vi "bufferFileManager.vi"(0 "Base Path (C:\\)":path=path "C:/", 1 "Write Limit (6000 writes)":i32=6000, 2 "Number of Files (7)":i32=7, 3 "Mode (Use)":enum16{"Init", "Use"}(ring)=enum."Use", 5 "Data Byte String (empty string)":string, 9 "Header Byte String (empty string)":string, 11 "Error In (no error)":errorcluster caption="Error In (No Error)", 12 "File Name Template (BUFFER_)":string="BUFFER_", 13 "File Extension (none)":string) -> (4 "refnums":refnum<file>[](array[refnum]), 6 "File Index":i32, 10 "Write Index":i32, 15 "Error Out":errorcluster)   [LabVIEW 2020]
doc: "This function manages a disk buffer located at the \"Base Path\". The number of buffer files is set by the \"Number of Files\" input, and they are labeled BUFFER_X by default where X is the zero-based buffer file number. BUFFER_ can be replaced in the file name by the user-specified \"File Name Template\". For each call to this function the \"Byte String\" data is written to the buffer files in turn. Files are created, cleared, and switched to as needed when the buffer \"Write Limit\" is met. If \"Byte String\" is empty nothing is written and the write counter is not incremented. To ignore the write limit or number of file limit, set these values to equal -1."
panel:
  # "NOTE: Mode is not necessary for use so it is disabled."
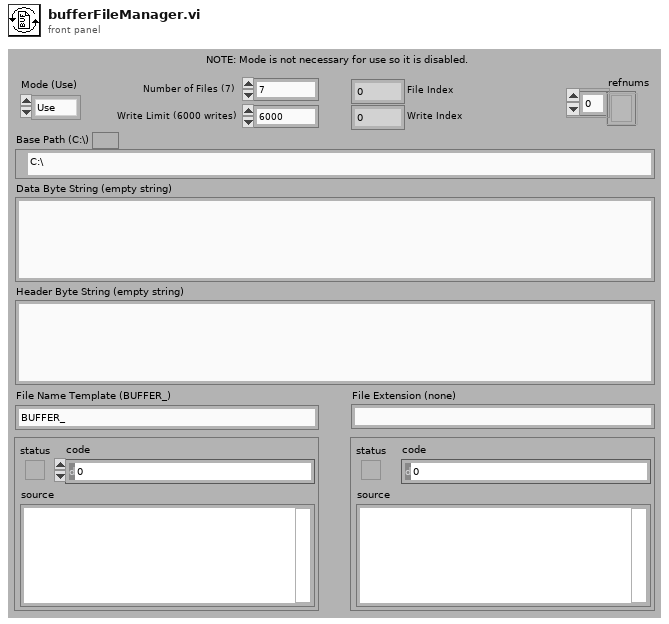
[diagram p1: front panel]
types:
  T1 = enum16{"open", "replace", "create", "open or create", "replace or create", "replace or create with confirmation"}
  T2 = cluster{"refnums":refnum<file>[], "File Index":i32, "Write Index":i32}
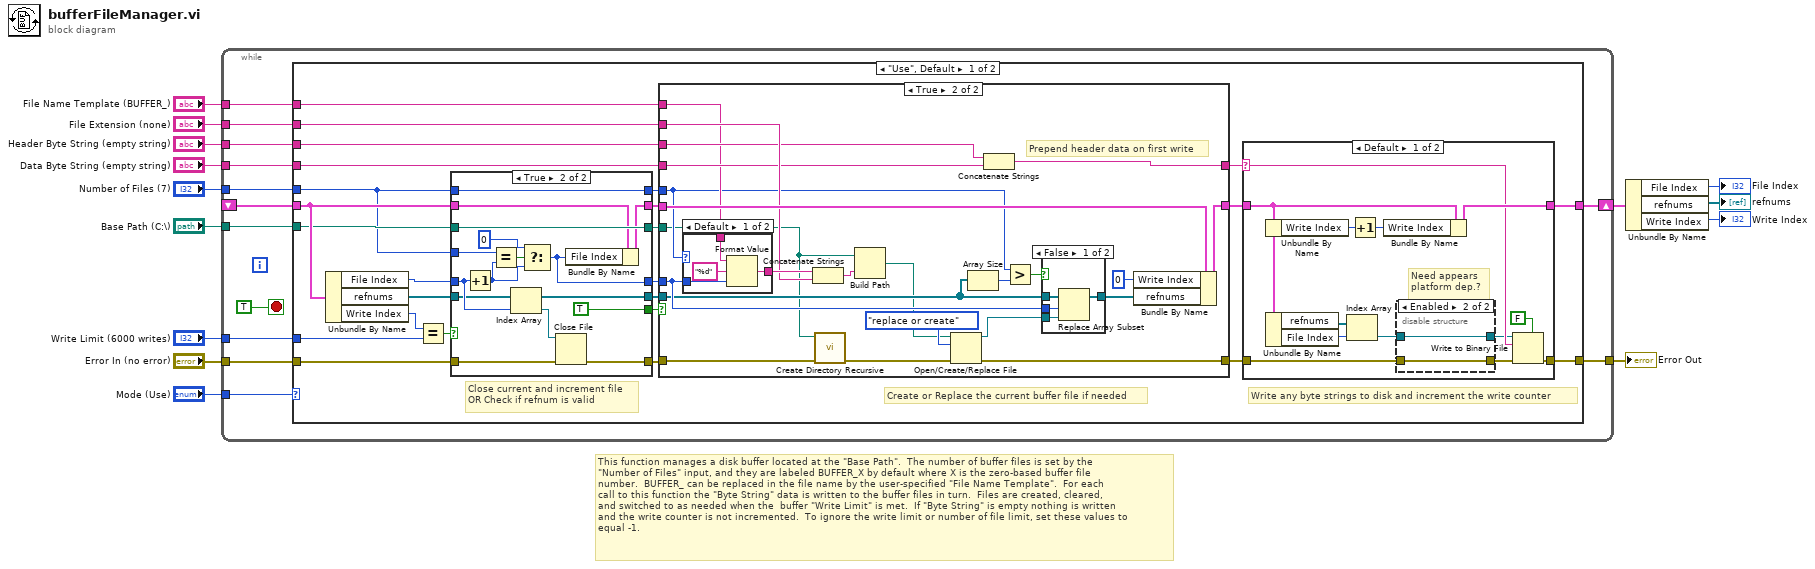
[diagram p0: block diagram]
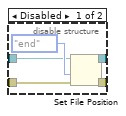
[diagram p2: hidden frame]
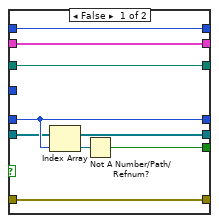
[diagram p4: hidden frame]
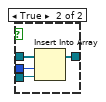
[diagram p7: hidden frame]
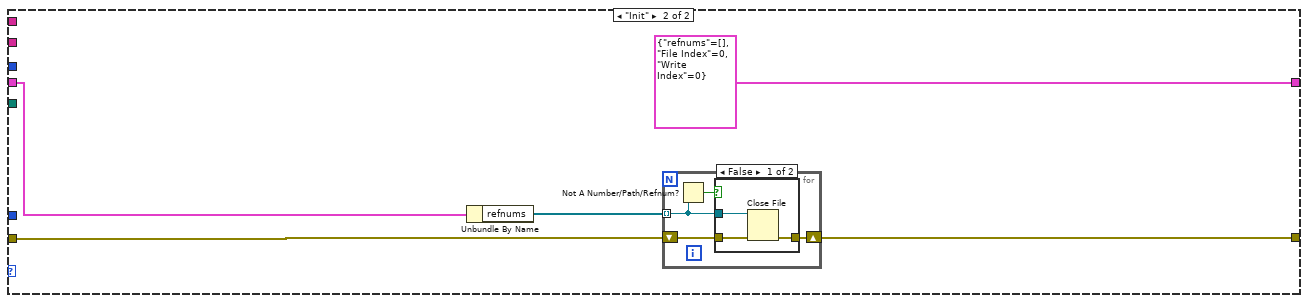
[diagram p8: hidden frame]
diagram:
  # "This function manages a disk buffer located at the \"Base Path\".  The number of buffer files is set by the \n\"Number of Files\" input, and they are labeled BUFFER_X by default where X is the zero-based buffer file \nnumber.  BUFFER_ can be replaced in the file name by the user-specified \"File Name Template\".  For each \ncall to this function the \"Byte String\" data is written to the buffer files in turn.  Files are created, cleared, \nand switched to as needed when the  buffer \"Write Limit\" is met.  If \"Byte String\" is empty nothing is written \nand the write counter is not incremented.  To ignore the write limit or number of file limit, set these values to \nequal -1."
  n1 = while {
    shift-right: [w25] -> w7
    shift-left: _ -> [w24]
    tunnel: "Number of Files (7)" -> [w22]
    tunnel: "Base Path (C:\\)" -> [w23]
    tunnel: "Error In (no error)" -> [w20]
    tunnel: "Write Limit (6000 writes)" -> [w21]
    tunnel: "Data Byte String (empty string)" -> [w26]
    tunnel: "Mode (Use)" -> [w19]
    tunnel: [w18] -> w8
    tunnel: "Header Byte String (empty string)" -> [w17]
    tunnel: "File Extension (none)" -> [w16]
    tunnel: "File Name Template (BUFFER_)" -> [w15]
    stop <- TRUE stop-if-true
    n2 = case shown="\"Use\", Default" w19 {
      tunnel: w26 -> [w31 _]
      tunnel: [w42 T2 {"refnums"=[], "File Index"=0, "Write Index"=0} ("USRs")] -> w25
      tunnel: w24 -> [w41 w138]
      tunnel: w23 -> [w40 _]
      tunnel: w22 -> [w36 _]
      tunnel: w21 -> [w39 _]
      tunnel: w20 -> [w38 w140]
      tunnel: [w37 w139] -> w18
      tunnel: w17 -> [w30 _]
      tunnel: w16 -> [w29 _]
      tunnel: w15 -> [w28 _]
      frame "Use", Default {
        # "Write any byte strings to disk and increment the write counter"
        # "Create or Replace the current buffer file if needed"
        # "Close current and increment file\nOR Check if refnum is valid"
        n3 = Unbundle By Name(w41) -> ("File Index"=w52:i32, "refnums"=w50:refnum<file>[], "Write Index"=w51:i32)
        n4 = Equal?(x=w51, y=w39) -> (x = y?=w47:bool)
        n5 = case shown="True" w47 {
          tunnel: w52 -> [w77 w94]
          tunnel: w50 -> [w76 w88]
          tunnel: [w81 TRUE] -> w49
          tunnel: w38 -> [w80 w93]
          tunnel: [w80 w92] -> w48
          tunnel: w40 -> [w78 w90]
          tunnel: w41 -> [w79 w86]
          tunnel: [w79 w85] -> w46
          tunnel: [w78 w90] -> w45
          tunnel: [w77 w84] -> w44
          tunnel: [w76 w88] -> w43
          tunnel: w36 -> [_ w97]
          tunnel: w36 -> [w75 w87]
          tunnel: [w75 w87] -> w35
          frame False {
            n6 = Index Array(array=w76, index=w77) -> (element=w82:refnum<file>)
            n7 = Not A Number/Path/Refnum?(number/path/refnum=w82) -> (NaN/Path/Refnum?=w81:bool)
          }
          frame True {
            n8 = Increment(x=w94) -> (x+1=w83:i32)
            n9 = Equal?(x=w97, y=w83) -> (x = y?=w96:bool)
            n10 = Index Array(array=w88, index=w94) -> (element=w91:refnum<file>)
            n11 = Select(t=0, s=w96, f=w83) -> (s? t:f=w84:i32)
            n12 = Close File(refnum=w91, error in=w93) -> (error out=w92:errorcluster)  [unwired: 1 out]
            n13 = Bundle By Name(cluster=w86, "File Index"=w84) -> (w85:T2)
          }
        }
        n14 = case shown="True" w49 {
          tunnel: w44 -> [_ w120]
          tunnel: w45 -> [_ w102]
          tunnel: w48 -> [w100 w104]
          tunnel: [w100 w122] -> w32
          tunnel: w46 -> [w99 w119]
          tunnel: [w99 w117] -> w33
          tunnel: w43 -> [_ w115]
          tunnel: w31 -> [w98 w108]
          tunnel: [w98 w109] -> w34
          tunnel: w35 -> [_ w105]
          tunnel: w30 -> [_ w107]
          tunnel: w29 -> [_ w110]
          tunnel: w28 -> [_ w106]
          frame False {
          }
          frame True {
            # "Prepend header data on first write"
            n15 = case shown="Default" w105 {
              tunnel: w120 -> [w126 _]
              tunnel: [w125 w128] -> w112
              tunnel: w106 -> [w124 w128]
              frame Default {
                n16 = Format Value(string ("")=w124, format string="%d", value (0)=w126) -> (output string=w125:string)
              }
              frame 1 {
              }
            }
            n17 = Concatenate Strings(w112, w110) -> (w111:string)
            n18 = call <vilib>:"Create Directory Recursive.vi"("error in (no error)"=w104, "directory"=w102) -> ("error out"=w103:errorcluster)  [unwired: 3 in, 2 out]
            n19 = Build Path(base path=w102, name or relative path=w111) -> (appended path=w101:path)
            n20 = Open/Create/Replace File(file path (use dialog)=w101, error in=w103, operation (0:open)=T1."replace or create") -> (refnum out=w121:refnum<file>, error out=w122:errorcluster)  [unwired: 3 in, 1 out]
            n21 = Array Size(array=w115) -> (size(s)=w114:i32)
            n22 = Concatenate Strings(w107, w108) -> (w109:string)
            n23 = Greater?(x=w105, y=w114) -> (0:w113:bool)
            n24 = case shown="False" w113 {
              tunnel: w121 -> [w132 w134]
              tunnel: w120 -> [w131 w135]
              tunnel: [w130 w133] -> w118
              tunnel: w115 -> [w129 w136]
              frame False {
                n25 = Replace Array Subset(array=w129, new element=w132, index=w131) -> (w130:refnum<file>[])
              }
              frame True {
                n26 = Insert Into Array(array=w136, index=w135, new element=w134) -> (w133:refnum<file>[])
              }
            }
            n27 = Bundle By Name(cluster=w119, "Write Index"=0, "refnums"=w118) -> (w117:T2)
          }
        }
        n28 = case shown="Default" w34 {
          selector: w34 -> [w61 _]
          tunnel: w32 -> [w60 w73]
          tunnel: w33 -> [w54 w74]
          tunnel: [w62 w74] -> w42
          tunnel: [w63 w73] -> w37
          frame Default {
            # "Need appears\nplatform dep.?"
            n29 = Unbundle By Name(w54) -> ("Write Index"=w53:i32)
            n30 = Unbundle By Name(w54) -> ("refnums"=w57:refnum<file>[], "File Index"=w56:i32)
            n31 = Index Array(array=w57, index=w56) -> (element=w55:refnum<file>)
            n32 = Increment(x=w53) -> (x+1=w64:i32)
            n33 = Bundle By Name(cluster=w54, "Write Index"=w64) -> (w62:T2)
            n34 = disable-structure shown="Enabled" {
              disable-tunnel: w60 -> [w70 w71]
              disable-tunnel: [w69 w71] -> w59
              disable-tunnel: [w67 w72] -> w58
              disable-tunnel: w55 -> [w66 w72]
              frame Disabled {
                n35 = Set File Position(refnum=w66, from (0:start)=enum16{"start", "end", "current"}."end", error in=w70) -> (refnum out=w67:refnum<file>, error out=w69:errorcluster)  [unwired: 1 in]
              }
              frame Enabled {
              }
            }
            n36 = Write to Binary File(file (use dialog)=w58, data=w61, error in=w59, 5:FALSE ("prepend array or string size? (T)")) -> (error out=w63:errorcluster)  [unwired: 2 in, 2 out]
          }
          frame "" {
          }
        }
      }
      frame "Init" {
        n37 = Unbundle By Name(w138) -> ("refnums"=w141:refnum<file>[])
        n38 = for {
          tunnel: w141 -> [w144] mode=indexing
          shift-right: [w142] -> w139
          shift-left: w140 -> [w143]
          n39 = Not A Number/Path/Refnum?(number/path/refnum=w144) -> (NaN/Path/Refnum?=w145:bool)
          n40 = case shown="False" w145 {
            tunnel: w144 -> [w148 _]
            tunnel: w143 -> [w147 w149]
            tunnel: [w146 w149] -> w142
            frame False {
              n41 = Close File(refnum=w148, error in=w147) -> (error out=w146:errorcluster)  [unwired: 1 out]
            }
            frame True {
            }
          }
        }
      }
    }
  }
  "Error Out" <- w8
  n42 = Unbundle By Name(w7) -> ("File Index"=→"File Index":i32, "refnums"=→"refnums":refnum<file>[], "Write Index"=→"Write Index":i32)
